vi "bats.parser.test.SequencedUnitHeader.Multiple.vi"() -> (3 "Passed":bool)   [LabVIEW 2022 SP3]
uses:
  Message.Spec.ctl
  pitch/MessageType.ctl
  pitch/AddOrderLong/AddOrderLong.Parameters.ctl
  pitch/Time/Time.Parameters.ctl
  pitch/SequencedUnitHeader/SequencedUnitHeader.Parameters.ctl
  pitch/SequencedUnitHeader/SequencedUnitHeader.lvclass
  pitch/PitchMessage/PitchMessage.lvclass
  pitch/Time/Time.lvclass
  pitch/AddOrderLong/AddOrderLong.lvclass
panel:
  in  "Expected Results":cluster{string[]}[](array[cluster])
  out "Results":cluster{string[]}[](array[cluster])
  out "Bytes.Out":u8[](array[numeric]) format="%.0x"
  out "Bytes.out (Visual)":u8[][](array[numeric]) format="%.0x"
  in  "Messages to Create":T1[](array[typedef])=[{"MessageType"=enum."AddOrderLong", "AddOrderLong.Parms"={"Time Offset"=447000, "Order Id"="ORID0001", "Side Indicator"="B", "Quantity"=20000, "Symbol"="AAPL", "Price"=0.905, "Add Flags"=1}, "Time.Parms"={"Seconds Since Midnight"=447000}, "SequencedUnitHeader.Parms"={"Hdr Count"=32, "Hdr Unit"=1, "Hdr Sequence"=1, "Starting Sequence"=1}}, {"MessageType"=enum."AddOrderLong", "AddOrderLong.Parms"={"Time Offset"=447000, "Order Id"="ORID0002", "Side Indicator"="B", "Quantity"=20000, "Symbol"="AAPL", "Price"=0.905, "Add Flags"=1}, "Time.Parms"={"Seconds Since Midnight"=447000}, "SequencedUnitHeader.Parms"={"Hdr Count"=32, "Hdr Unit"=1, "Hdr Sequence"=1, "Starting Sequence"=1}}, {"MessageType"=enum."AddOrderLong", "AddOrderLong.Parms"={"Time Offset"=447000, "Order Id"="ORID0003", "Side Indicator"="B", "Quantity"=20000, "Symbol"="AAPL", "Price"=0.905, "Add Flags"=1}, "Time.Parms"={"Seconds Since Midnight"=447000}, "SequencedUnitHeader.Parms"={"Hdr Count"=32, "Hdr Unit"=1, "Hdr Sequence"=1, "Starting Sequence"=1}}, {"MessageType"=enum."AddOrderLong", "AddOrderLong.Parms"={"Time Offset"=447000, "Order Id"="ORID0004", "Side Indicator"="B", "Quantity"=20000, "Symbol"="AAPL", "Price"=0.905, "Add Flags"=1}, "Time.Parms"={"Seconds Since Midnight"=447000}, "SequencedUnitHeader.Parms"={"Hdr Count"=32, "Hdr Unit"=1, "Hdr Sequence"=1, "Starting Sequence"=1}}, {"MessageType"=enum."AddOrderLong", "AddOrderLong.Parms"={"Time Offset"=447000, "Order Id"="ORID0005", "Side Indicator"="B", "Quantity"=20000, "Symbol"="AAPL", "Price"=0.905, "Add Flags"=1}, "Time.Parms"={"Seconds Since Midnight"=447000}, "SequencedUnitHeader.Parms"={"Hdr Count"=32, "Hdr Unit"=1, "Hdr Sequence"=1, "Starting Sequence"=1}}, {"MessageType"=enum."AddOrderLong", "AddOrderLong.Parms"={"Time Offset"=447000, "Order Id"="ORID0006", "Side Indicator"="B", "Quantity"=20000, "Symbol"="AAPL", "Price"=0.905, "Add Flags"=1}, "Time.Parms"={"Seconds Since Midnight"=447000}, "SequencedUnitHeader.Parms"={"Hdr Count"=32, "Hdr Unit"=1, "Hdr Sequence"=1, "Starting Sequence"=1}}, {"MessageType"=enum."AddOrderLong", "AddOrderLong.Parms"={"Time Offset"=447000, "Order Id"="ORID0007", "Side Indicator"="B", "Quantity"=20000, "Symbol"="AAPL", "Price"=0.905, "Add Flags"=1}, "Time.Parms"={"Seconds Since Midnight"=447000}, "SequencedUnitHeader.Parms"={"Hdr Count"=32, "Hdr Unit"=1, "Hdr Sequence"=1, "Starting Sequence"=1}}, {"MessageType"=enum."AddOrderLong", "AddOrderLong.Parms"={"Time Offset"=447000, "Order Id"="ORID0008", "Side Indicator"="B", "Quantity"=20000, "Symbol"="AAPL", "Price"=0.905, "Add Flags"=1}, "Time.Parms"={"Seconds Since Midnight"=447000}, "SequencedUnitHeader.Parms"={"Hdr Count"=32, "Hdr Unit"=1, "Hdr Sequence"=1, "Starting Sequence"=1}}, {"MessageType"=enum."AddOrderLong", "AddOrderLong.Parms"={"Time Offset"=447000, "Order Id"="ORID0009", "Side Indicator"="B", "Quantity"=20000, "Symbol"="AAPL", "Price"=0.905, "Add Flags"=1}, "Time.Parms"={"Seconds Since Midnight"=447000}, "SequencedUnitHeader.Parms"={"Hdr Count"=32, "Hdr Unit"=1, "Hdr Sequence"=1, "Starting Sequence"=1}}, {"MessageType"=enum."AddOrderLong", "AddOrderLong.Parms"={"Time Offset"=447000, "Order Id"="ORID000A", "Side Indicator"="B", "Quantity"=20000, "Symbol"="AAPL", "Price"=0.905, "Add Flags"=1}, "Time.Parms"={"Seconds Since Midnight"=447000}, "SequencedUnitHeader.Parms"={"Hdr Count"=32, "Hdr Unit"=1, "Hdr Sequence"=1, "Starting Sequence"=1}}, {"MessageType"=enum."AddOrderLong", "AddOrderLong.Parms"={"Time Offset"=447000, "Order Id"="ORID000B", "Side Indicator"="B", "Quantity"=20000, "Symbol"="AAPL", "Price"=0.905, "Add Flags"=1}, "Time.Parms"={"Seconds Since Midnight"=447000}, "SequencedUnitHeader.Parms"={"Hdr Count"=32, "Hdr Unit"=1, "Hdr Sequence"=1, "Starting Sequence"=1}}]
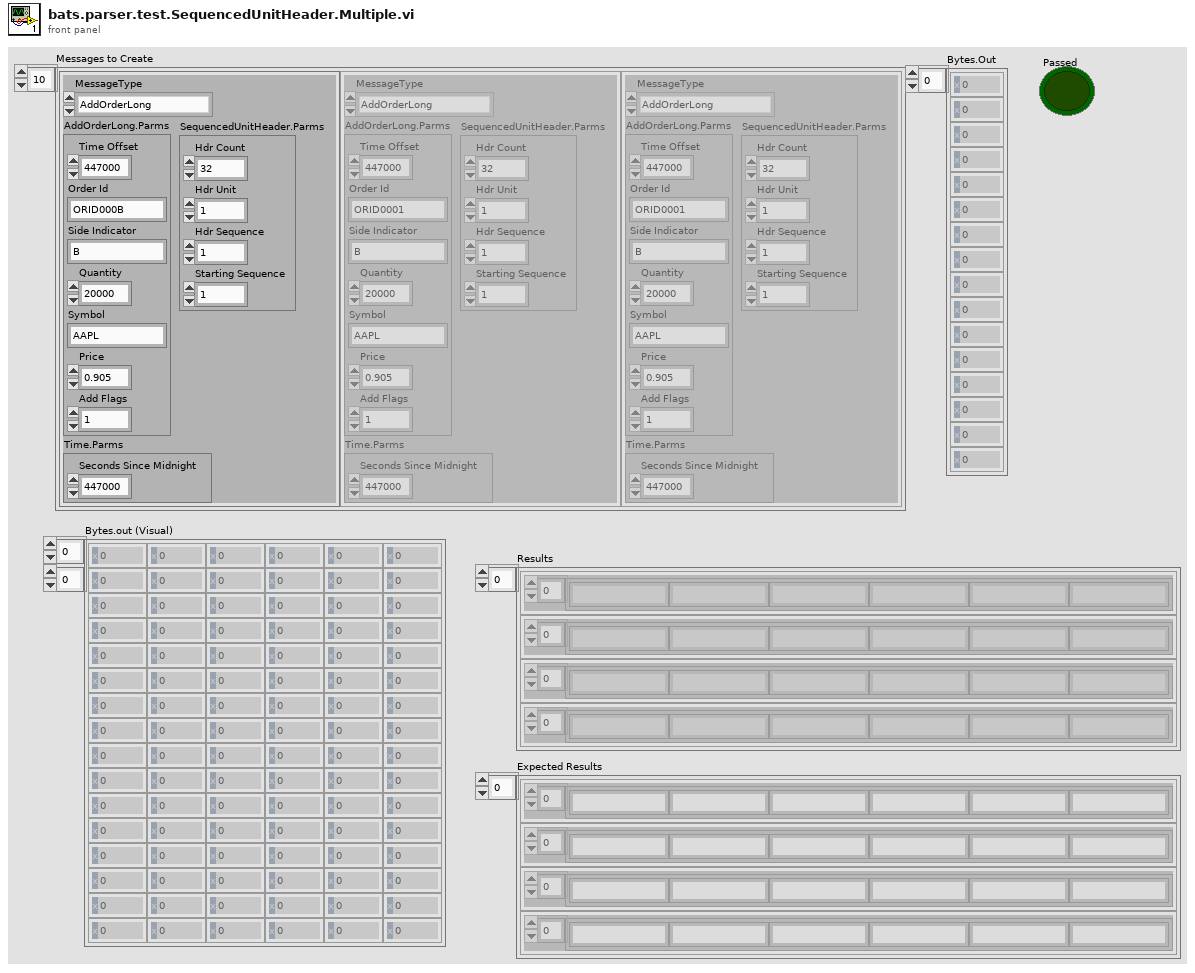
[diagram p1: front panel]
types:
  T1 = typedef "Message.Spec.ctl" = cluster{"MessageType":T2, "AddOrderLong.Parms":T3, "Time.Parms":T4, "SequencedUnitHeader.Parms":T5}
  T2 = typedef "MessageType.ctl" = enum16{"SequencedUnitHeader", "AddOrderLong", "AddOrderShort", "AddOrderExpanded", "Time"}
  T3 = typedef "AddOrderLong.lvclass/AddOrderLong.Parameters.ctl" = cluster{"Time Offset":u32, "Order Id":string, "Side Indicator":string, "Quantity":u32, "Symbol":string, "Price":dbl, "Add Flags":u8}
  T4 = typedef "Time.lvclass/Time.Parameters.ctl" = cluster{"Seconds Since Midnight":u32}
  T5 = typedef "SequencedUnitHeader.lvclass/SequencedUnitHeader.Parameters.ctl" = cluster{"Hdr Count":u8, "Hdr Unit":u8, "Hdr Sequence":u32, "Starting Sequence":u32}
  T6 = typedef "FieldValue.ctl" = variant
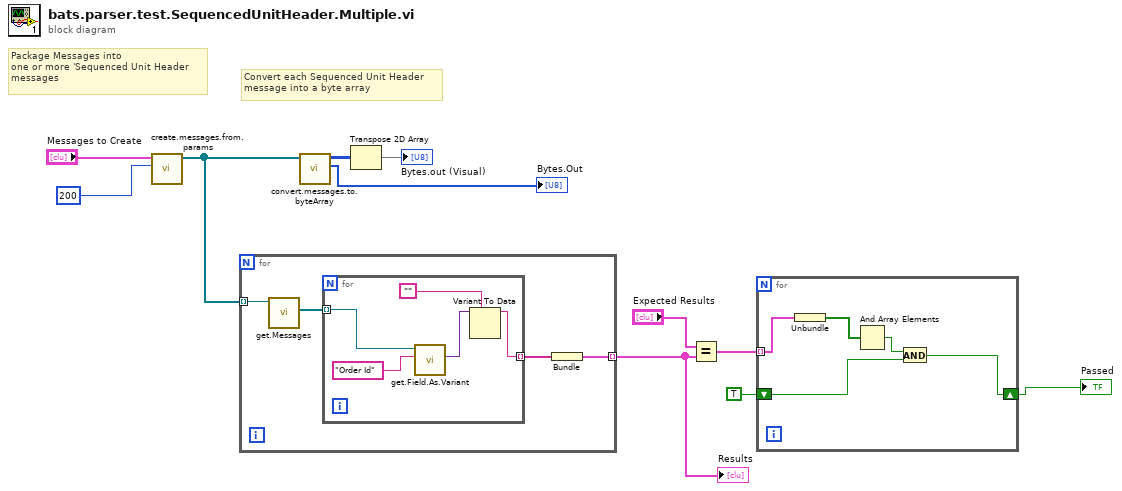
[diagram p0: block diagram]
diagram:
  # "Convert each Sequenced Unit Header\nmessage into a byte array"
  # "Package Messages into\none or more 'Sequenced Unit Header\nmessages"
  n1 = call "create.messages.from.params.vi"("Max.Frame.Size"=u16 200, "Messages to Create"="Messages to Create") -> ("Messages.Out"=w6:refnum<class "SequencedUnitHeader.lvclass">[])  [unwired: 9 in]
  n2 = for {
    tunnel: w6 -> [w15] mode=indexing
    tunnel: [w12] -> w5 mode=indexing
    n3 = call-dynamic "get.Messages.vi"("SequencedUnitHeader in"=w15) -> ("Messages.Out"=w14:refnum<class "PitchMessage.lvclass">[])  [unwired: 8 in, 2 out]
    n4 = for {
      tunnel: w14 -> [w20] mode=indexing
      tunnel: [w16] -> w13 mode=indexing
      n5 = call-dynamic "get.Field.As.Variant.vi"("Field.Name"="Order Id", "PitchMessage in"=w20) -> ("Value.Variant"=w18:T6)  [unwired: 7 in, 2 out]
      n6 = Variant To Data(type="", Variant=w18) -> (data=w16:string)  [unwired: 1 in, 1 out]
    }
    n7 = Bundle(w13) -> (w12:cluster{string[]})  [unwired: 1 in]
  }
  "Results" <- w5
  n8 = call "convert.messages.to.byteArray.vi"("Messages.In"=w6) -> ("ByteArray.out"=→"Bytes.Out":u8[], "2D.ByteArray.out"=w9:u8[][])  [unwired: 9 in]
  n9 = Transpose 2D Array(2D array=w9) -> (transposed array=→"Bytes.out (Visual)":u8[][])
  n10 = Equal?(x="Expected Results", y=w5) -> (x = y?=w3:cluster{bool[]}[])
  n11 = for {
    tunnel: w3 -> [w25] mode=indexing
    shift-right: [w22] -> w1
    shift-left: TRUE -> [w23]
    n12 = Unbundle(w25) -> (w24:bool[])
    n13 = And Array Elements(Boolean array=w24) -> (logical AND=w21:bool)
    n14 = And(x=w21, y=w23) -> (x .and. y?=w22:bool)
  }
  "Passed" <- w1
